vi "Test Alias.vi"() -> ()   [LabVIEW 2020]
uses:
  VisaResource/VisaResource.lvclass
  C:/dev/Vireo/PicoG/PicoG-Processor/PicoG-Core/DeployResource/DeployResource.lvclass
  DeployResource/DeployResource.lvclass
  C:/dev/Vireo/PicoG/PicoG-Processor/PicoG-Core/VisaResource/VisaResource.lvclass
panel:
  out "Old Alias":string
  in  "New Alias (Unchanged)":string
  out "error out":errorcluster
  out "Alias":string
  in  "VISA resource name":refnum<visa-resource-name>
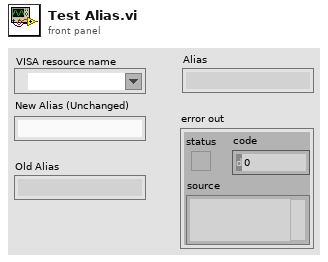
[diagram p1: front panel]
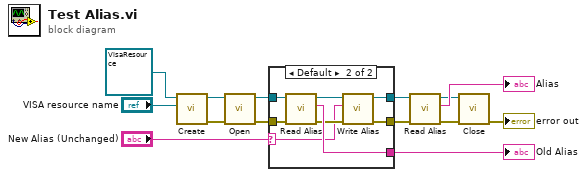
[diagram p0: block diagram]
diagram:
  n1 = call-dynamic "Create.vi"("Resource"="VISA resource name", "VisaResource in"=refnum<class "VisaResource.lvclass"> refnum) -> ("error out"=w11:errorcluster, "VisaResource out"=w12:refnum<class "VisaResource.lvclass">)  [unwired: 8 in]
  n2 = call-dynamic "Open.vi"("error in (no error)"=w11, "VisaResource in"=w12) -> ("error out"=w2:errorcluster, "VisaResource out"=w5:refnum<class "VisaResource.lvclass">)  [unwired: 8 in]
  n3 = case shown="Default" "New Alias (Unchanged)" {
    selector: "New Alias (Unchanged)" -> [_ w19]
    tunnel: w5 -> [w16 w24]
    tunnel: [w16 w18] -> w4
    tunnel: [w15 w17] -> w3
    tunnel: w2 -> [w15 w23]
    tunnel: [_ w22] -> w1
    frame "" {
    }
    frame Default {
      n4 = call "Read Alias.vi"("error in (no error)"=w23, "DeployResource in"=w24) -> ("error out"=w20:errorcluster, "Alias"=w22:string, "DeployResource out"=w21:refnum<class "VisaResource.lvclass">)  [unwired: 7 in]
      n5 = call "Write Alias.vi"("error in (no error)"=w20, "Alias"=w19, "DeployResource in"=w21) -> ("error out"=w17:errorcluster, "DeployResource out"=w18:refnum<class "VisaResource.lvclass">)  [unwired: 7 in]
    }
  }
  "Old Alias" <- w1
  n6 = call "Read Alias.vi"("error in (no error)"=w3, "DeployResource in"=w4) -> ("error out"=w8:errorcluster, "Alias"=→"Alias":string, "DeployResource out"=w9:refnum<class "VisaResource.lvclass">)  [unwired: 7 in]
  n7 = call-dynamic "Close.vi"("error in (no error)"=w8, "VisaResource in"=w9) -> ("error out"=→"error out":errorcluster)  [unwired: 8 in, 1 out]
